vi "力特性判定.vi"(0 "曲线引用":refnum<vi>, 1 "力特性判定条件":T1, 3 "错误输入":errorcluster) -> (5 "曲线引用输出":refnum<vi>, 6 "OK？":bool, 8 "错误输出":errorcluster)   [LabVIEW 2019]
uses:
  Global_Variable/A131258.vi
  Global_Variable/Global.vi
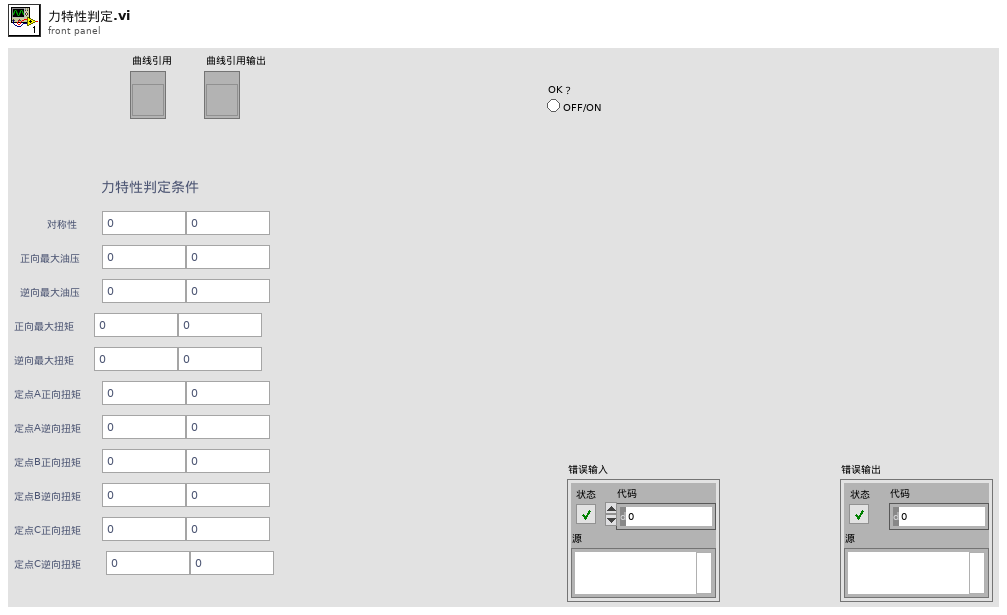
[diagram p1: front panel]
types:
  T1 = cluster{"           对称性":cluster{"下限":dbl, "上限":dbl}, "  正向最大油压":cluster{"下限":dbl, "上限":dbl}, "  逆向最大油压":cluster{"下限":dbl, "上限":dbl}, "正向最大扭矩":cluster{"下限":dbl, "上限":dbl}, "逆向最大扭矩":cluster{"下限":dbl, "上限":dbl}, "定点A正向扭矩":cluster{"下限":dbl, "上限":dbl}, "定点A逆向扭矩":cluster{"下限":dbl, "上限":dbl}, "定点B正向扭矩":cluster{"下限":dbl, "上限":dbl}, "定点B逆向扭矩":cluster{"下限":dbl, "上限":dbl}, "定点C正向扭矩":cluster{"下限":dbl, "上限":dbl}, "定点C逆向扭矩 ":cluster{"下限":dbl, "上限":dbl}}
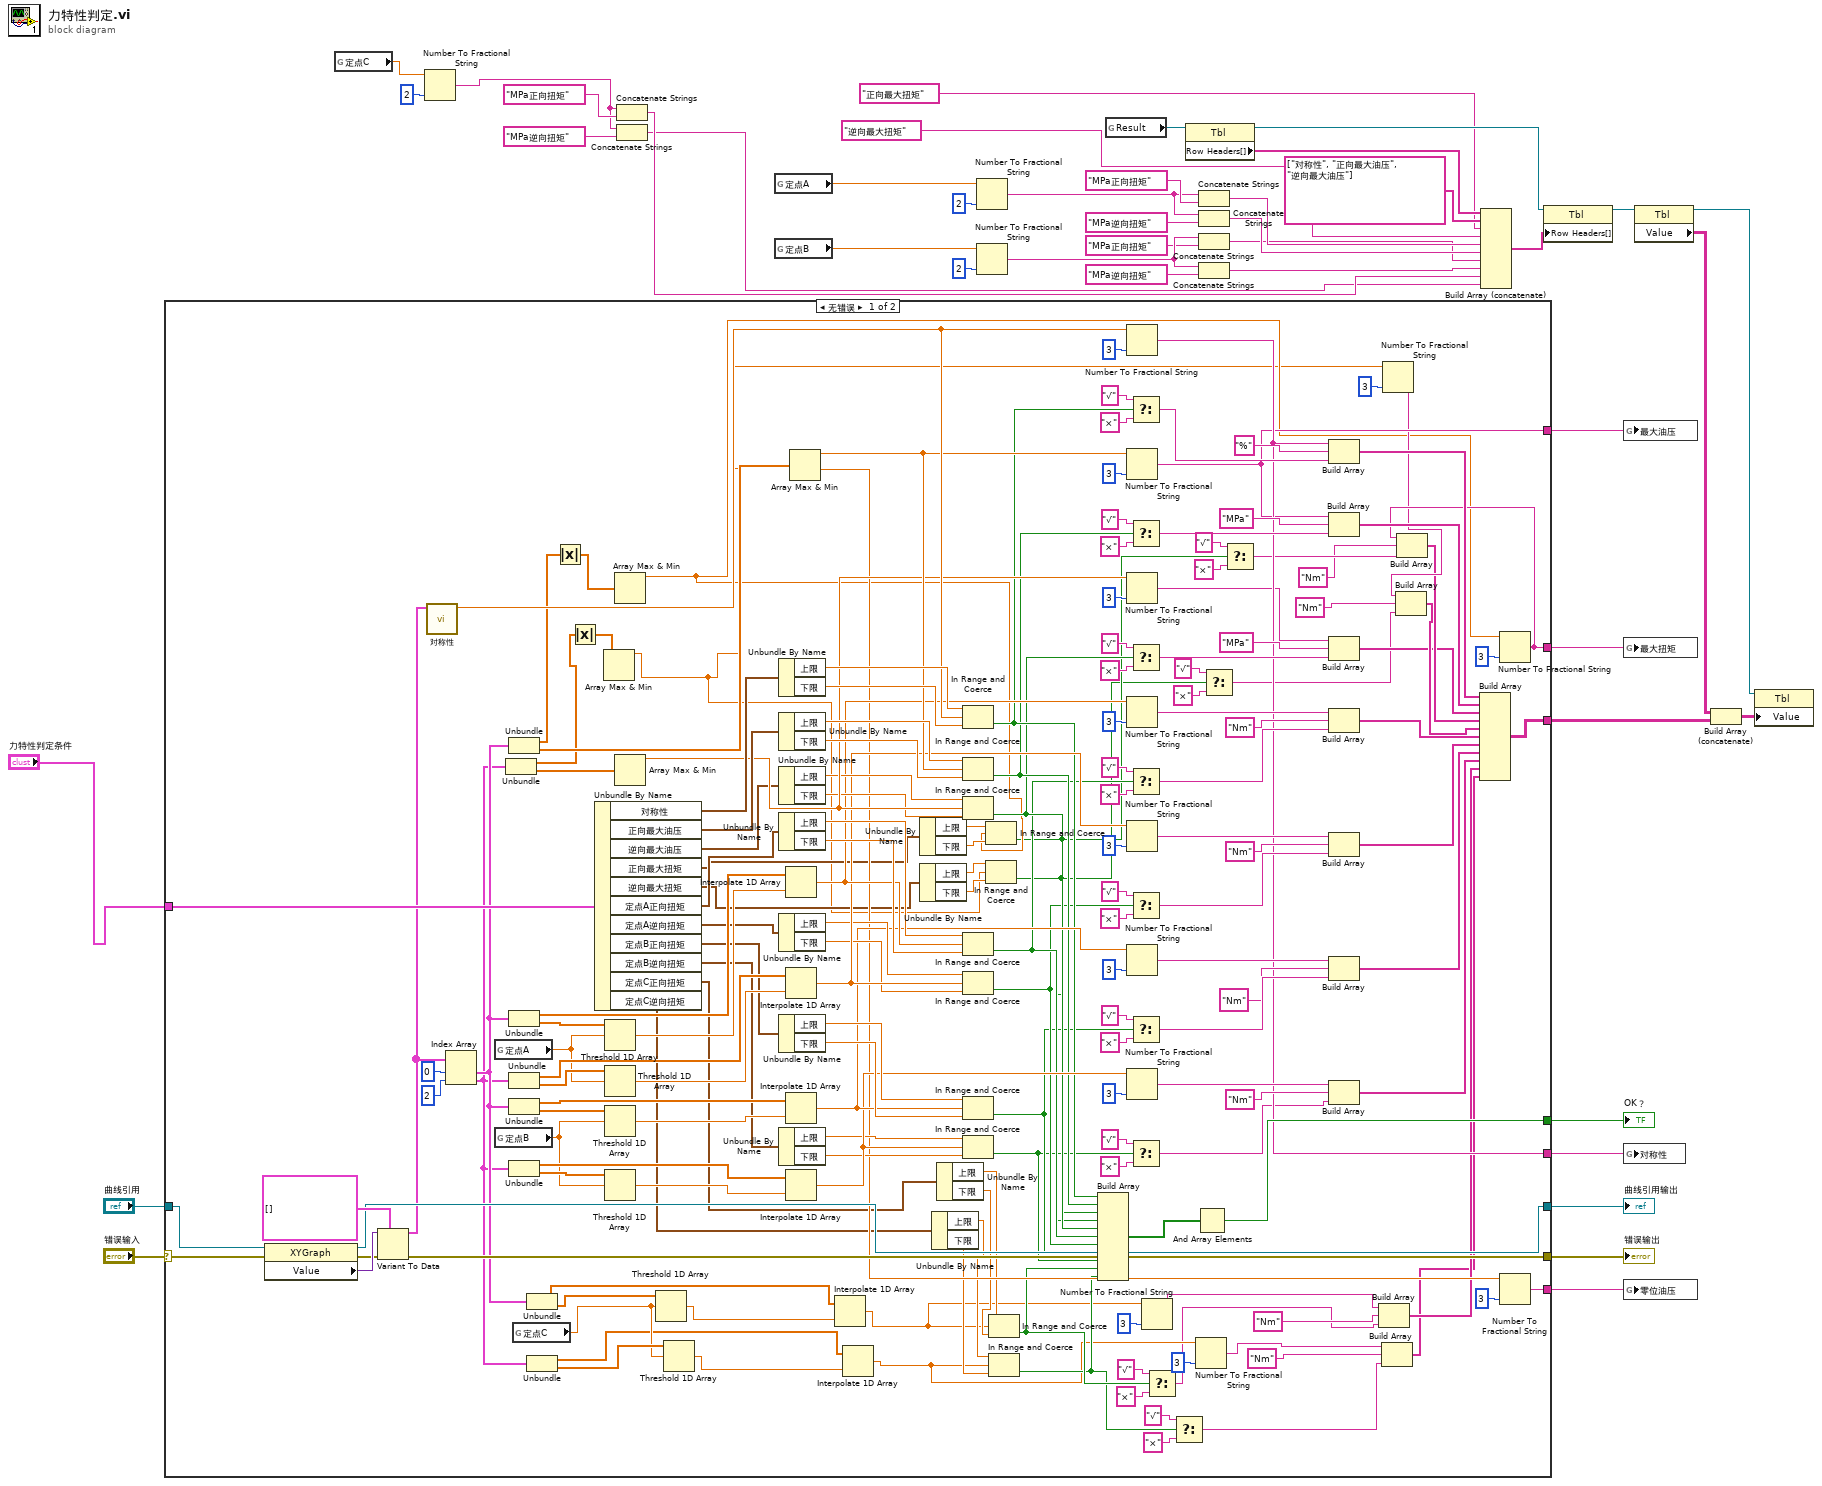
[diagram p0: block diagram]
diagram:
  n1 = case shown="无错误" "错误输入" {
    selector: "错误输入" -> [w219 w223]
    tunnel: [w216 w223] -> w42
    tunnel: "曲线引用" -> [w215 w222]
    tunnel: [w218 w222] -> w40
    tunnel: [w122 _] -> w39
    tunnel: "力特性判定条件" -> [w214 _]
    tunnel: [w121 _] -> w35
    tunnel: [w116 _] -> w14
    tunnel: [w115 _] -> w13
    tunnel: [w102 _] -> w12
    tunnel: [w111 _] -> w11
    frame No Error {
      n2 = property class="XYGraph"(reference=w215, error in=w219) -> (reference out=w218:refnum<vi>, error out=w217:errorcluster, "Value"=w221:variant)
      n3 = Variant To Data(error in=w217, type=cluster{dbl[], dbl[]}[] [], Variant=w221) -> (data=w204:cluster{dbl[], dbl[]}[], error out=w216:errorcluster)
      n4 = call "对称性.vi"("XY图"=w204) -> ("对称性"=w210:dbl)  [unwired: 8 in, 2 out]
      n5 = Index Array(array=w204, index #1=0 ("索引"), index #2=2 ("索引")) -> (element #1=w90:cluster{dbl[], dbl[]}, element #2=w89:cluster{dbl[], dbl[]})
      n6 = global read "A131258.vi" "定点A"() -> (w118:dbl)
      n7 = global read "A131258.vi" "定点B"() -> (w117:dbl)
      n8 = Unbundle(w89) -> (w47:dbl[], w119:dbl[])
      n9 = Unbundle(w90) -> (w45:dbl[], w120:dbl[])
      n10 = Unbundle(w90) -> (w176:dbl[], w177:dbl[])
      n11 = Unbundle(w89) -> (w171:dbl[], w170:dbl[])
      n12 = Unbundle(w90) -> (w152:dbl[], w153:dbl[])
      n13 = Unbundle(w89) -> (w145:dbl[], w144:dbl[])
      n14 = global read "A131258.vi" "定点C"() -> (w86:dbl)
      n15 = Unbundle(w90) -> (w83:dbl[], w88:dbl[])
      n16 = Unbundle(w89) -> (w82:dbl[], w87:dbl[])
      n17 = Absolute Value(x=w45) -> (abs(x)=w44:dbl[])
      n18 = Absolute Value(x=w47) -> (abs(x)=w48:dbl[])
      n19 = Unbundle By Name(w214) -> ("对称性"=w213:cluster{"下限":dbl, "上限":dbl}, "正向最大油压"=w196:cluster{"下限":dbl, "上限":dbl}, "逆向最大油压"=w186:cluster{"下限":dbl, "上限":dbl}, "正向最大扭矩"=w99:cluster{"下限":dbl, "上限":dbl}, "逆向最大扭矩"=w98:cluster{"下限":dbl, "上限":dbl}, "定点A正向扭矩"=w107:cluster{"下限":dbl, "上限":dbl}, "定点A逆向扭矩"=w108:cluster{"下限":dbl, "上限":dbl}, "定点B正向扭矩"=w109:cluster{"下限":dbl, "上限":dbl}, "定点B逆向扭矩"=w110:cluster{"下限":dbl, "上限":dbl}, "定点C正向扭矩"=w81:cluster{"下限":dbl, "上限":dbl}, "定点C逆向扭矩"=w80:cluster{"下限":dbl, "上限":dbl})
      n20 = Array Max & Min(array=w48) -> (max value=w46:dbl)  [unwired: 3 out]
      n21 = Threshold 1D Array(2:w118, 3:w177) -> (0:w175:dbl)  [unwired: 1 in]
      n22 = Threshold 1D Array(2:w118, 3:w170) -> (0:w172:dbl)  [unwired: 1 in]
      n23 = Threshold 1D Array(2:w117, 3:w153) -> (0:w151:dbl)  [unwired: 1 in]
      n24 = Threshold 1D Array(2:w117, 3:w144) -> (0:w146:dbl)  [unwired: 1 in]
      n25 = Array Max & Min(array=w44) -> (max value=w93:dbl)  [unwired: 3 out]
      n26 = Array Max & Min(array=w119) -> (max value=w194:dbl)  [unwired: 3 out]
      n27 = Threshold 1D Array(2:w86, 3:w88) -> (0:w85:dbl)  [unwired: 1 in]
      n28 = Threshold 1D Array(2:w86, 3:w87) -> (0:w84:dbl)  [unwired: 1 in]
      n29 = Unbundle By Name(w213) -> ("上限"=w212:dbl, "下限"=w211:dbl)
      n30 = Unbundle By Name(w196) -> ("上限"=w197:dbl, "下限"=w198:dbl)
      n31 = Unbundle By Name(w186) -> ("上限"=w193:dbl, "下限"=w192:dbl)
      n32 = Unbundle By Name(w107) -> ("上限"=w178:dbl, "下限"=w179:dbl)
      n33 = Unbundle By Name(w108) -> ("上限"=w169:dbl, "下限"=w168:dbl)
      n34 = Unbundle By Name(w109) -> ("上限"=w154:dbl, "下限"=w155:dbl)
      n35 = Unbundle By Name(w110) -> ("上限"=w143:dbl, "下限"=w142:dbl)
      n36 = Interpolate 1D Array(1:w175, 2:w176) -> (0:w174:dbl)
      n37 = Interpolate 1D Array(1:w172, 2:w171) -> (0:w173:dbl)
      n38 = Interpolate 1D Array(1:w151, 2:w152) -> (0:w150:dbl)
      n39 = Interpolate 1D Array(1:w146, 2:w145) -> (0:w147:dbl)
      n40 = Array Max & Min(array=w120) -> (max value=w195:dbl, min value=w112:dbl)  [unwired: 2 out]
      n41 = Interpolate 1D Array(1:w85, 2:w83) -> (0:w64:dbl)
      n42 = Interpolate 1D Array(1:w84, 2:w82) -> (0:w65:dbl)
      n43 = Unbundle By Name(w99) -> ("上限"=w97:dbl, "下限"=w96:dbl)
      n44 = Unbundle By Name(w98) -> ("上限"=w95:dbl, "下限"=w94:dbl)
      n45 = Unbundle By Name(w80) -> ("上限"=w77:dbl, "下限"=w76:dbl)
      n46 = Unbundle By Name(w81) -> ("上限"=w79:dbl, "下限"=w78:dbl)
      n47 = In Range and Coerce(upper limit=w212, x=w210, lower limit=w211) -> (In Range?=w135:bool)  [unwired: 1 out]
      n48 = In Range and Coerce(upper limit=w197, x=w195, lower limit=w198) -> (In Range?=w133:bool)  [unwired: 1 out]
      n49 = In Range and Coerce(upper limit=w193, x=w194, lower limit=w192) -> (In Range?=w132:bool)  [unwired: 1 out]
      n50 = In Range and Coerce(upper limit=w178, x=w174, lower limit=w179) -> (In Range?=w130:bool)  [unwired: 1 out]
      n51 = In Range and Coerce(upper limit=w169, x=w173, lower limit=w168) -> (In Range?=w128:bool)  [unwired: 1 out]
      n52 = In Range and Coerce(upper limit=w154, x=w150, lower limit=w155) -> (In Range?=w126:bool)  [unwired: 1 out]
      n53 = In Range and Coerce(upper limit=w143, x=w147, lower limit=w142) -> (In Range?=w124:bool)  [unwired: 1 out]
      n54 = In Range and Coerce(upper limit=w97, x=w93, lower limit=w96) -> (In Range?=w92:bool)  [unwired: 1 out]
      n55 = In Range and Coerce(upper limit=w95, x=w46, lower limit=w94) -> (In Range?=w91:bool)  [unwired: 1 out]
      n56 = In Range and Coerce(upper limit=w79, x=w64, lower limit=w78) -> (In Range?=w71:bool)  [unwired: 1 out]
      n57 = In Range and Coerce(upper limit=w77, x=w65, lower limit=w76) -> (In Range?=w70:bool)  [unwired: 1 out]
      n58 = Build Array(w135, w133, w92, w91, w132, w130, w128, w126, w124, w71, w70) -> (w123:bool[])
      n59 = Number To Fractional String(number=w210, precision (6)=i16 3 ("精度(6)")) -> (F-format string=w116:string)  [unwired: 2 in]
      n60 = Number To Fractional String(number=w195, precision (6)=i16 3 ("精度(6)")) -> (F-format string=w115:string)  [unwired: 2 in]
      n61 = Number To Fractional String(number=w194, precision (6)=i16 3 ("精度(6)")) -> (F-format string=w60:string)  [unwired: 2 in]
      n62 = Number To Fractional String(number=w174, precision (6)=i16 3 ("精度(6)")) -> (F-format string=w181:string)  [unwired: 2 in]
      n63 = Number To Fractional String(number=w173, precision (6)=i16 3 ("精度(6)")) -> (F-format string=w166:string)  [unwired: 2 in]
      n64 = Number To Fractional String(number=w150, precision (6)=i16 3 ("精度(6)")) -> (F-format string=w157:string)  [unwired: 2 in]
      n65 = Number To Fractional String(number=w147, precision (6)=i16 3 ("精度(6)")) -> (F-format string=w140:string)  [unwired: 2 in]
      n66 = Select(t="√" ("元素"), s=w135, f="×" ("元素")) -> (s? t:f=w205:string)
      n67 = Select(t="√" ("元素"), s=w133, f="×" ("元素")) -> (s? t:f=w203:string)
      n68 = Select(t="√" ("元素"), s=w132, f="×" ("元素")) -> (s? t:f=w187:string)
      n69 = Select(t="√" ("元素"), s=w130, f="×" ("元素")) -> (s? t:f=w185:string)
      n70 = Select(t="√" ("元素"), s=w128, f="×" ("元素")) -> (s? t:f=w162:string)
      n71 = Select(t="√" ("元素"), s=w126, f="×" ("元素")) -> (s? t:f=w161:string)
      n72 = Select(t="√" ("元素"), s=w124, f="×" ("元素")) -> (s? t:f=w49:string)
      n73 = Number To Fractional String(number=w64, precision (6)=i16 3 ("精度(6)")) -> (F-format string=w67:string)  [unwired: 2 in]
      n74 = Select(t="√" ("元素"), s=w71, f="×" ("元素")) -> (s? t:f=w50:string)
      n75 = Select(t="√" ("元素"), s=w70, f="×" ("元素")) -> (s? t:f=w52:string)
      n76 = Number To Fractional String(number=w65, precision (6)=i16 3 ("精度(6)")) -> (F-format string=w66:string)  [unwired: 2 in]
      n77 = And Array Elements(Boolean array=w123) -> (logical AND=w122:bool)
      n78 = Select(t="√" ("元素"), s=w91, f="×" ("元素")) -> (s? t:f=w54:string)
      n79 = Select(t="√" ("元素"), s=w92, f="×" ("元素")) -> (s? t:f=w57:string)
      n80 = Build Array(w116, "%" ("元素"), w205) -> (w136:string[])
      n81 = Build Array(w115, "MPa" ("元素"), w203) -> (w134:string[])
      n82 = Build Array(w60, "MPa" ("元素"), w187) -> (w61:string[])
      n83 = Build Array(w181, "Nm" ("元素"), w185) -> (w131:string[])
      n84 = Build Array(w166, "Nm" ("元素"), w162) -> (w129:string[])
      n85 = Build Array(w157, "Nm" ("元素"), w161) -> (w127:string[])
      n86 = Build Array(w140, "Nm" ("元素"), w49) -> (w125:string[])
      n87 = Build Array(w67, "Nm" ("元素"), w50) -> (w59:string[])
      n88 = Build Array(w66, "Nm" ("元素"), w52) -> (w58:string[])
      n89 = Number To Fractional String(number=w46, precision (6)=i16 3 ("精度(6)")) -> (F-format string=w100:string)  [unwired: 2 in]
      n90 = Build Array(w100, "Nm" ("元素"), w54) -> (w63:string[])
      n91 = Number To Fractional String(number=w93, precision (6)=i16 3 ("精度(6)")) -> (F-format string=w102:string)  [unwired: 2 in]
      n92 = Build Array(w102, "Nm" ("元素"), w57) -> (w62:string[])
      n93 = Build Array(w136, w134, w61, w62, w63, w131, w129, w127, w125, w59, w58) -> (w121:string[][])
      n94 = Number To Fractional String(number=w112, precision (6)=i16 3 ("精度(6)")) -> (F-format string=w111:string)  [unwired: 2 in]
    }
    frame Error {
    }
  }
  "错误输出" <- w42
  "曲线引用输出" <- w40
  "OK？" <- w39
  n95 = global read "A131258.vi" "定点C"() -> (w6:dbl)
  n96 = Number To Fractional String(number=w6, precision (6)=i16 2 ("精度(6)")) -> (F-format string=w3:string)  [unwired: 2 in]
  n97 = Concatenate Strings(w3, "MPa正向扭矩") -> (w2:string)
  n98 = Concatenate Strings(w3, "MPa逆向扭矩") -> (w1:string)
  n99 = global read "A131258.vi" "定点A"() -> (w28:dbl)
  n100 = global read "A131258.vi" "定点B"() -> (w27:dbl)
  n101 = Number To Fractional String(number=w28, precision (6)=i16 2 ("精度(6)")) -> (F-format string=w25:string)  [unwired: 2 in]
  n102 = Number To Fractional String(number=w27, precision (6)=i16 2 ("精度(6)")) -> (F-format string=w22:string)  [unwired: 2 in]
  n103 = global read "Global.vi" "Result"() -> (w34:refnum<vi>)
  n104 = property class="Tbl"(reference=w34) -> (reference out=w33:refnum<vi>, "Row Headers[]"=w31:string[])  [unwired: 1 in, 1 out]
  n105 = Concatenate Strings(w25, "MPa正向扭矩") -> (w20:string)
  n106 = Concatenate Strings(w25, "MPa逆向扭矩") -> (w19:string)
  n107 = Concatenate Strings(w22, "MPa正向扭矩") -> (w18:string)
  n108 = Concatenate Strings(w22, "MPa逆向扭矩") -> (w17:string)
  n109 = Build Array (concatenate)(w31, string[] ["对称性", "正向最大油压", "逆向最大油压"] ("列首字符串[]"), "正向最大扭矩", "逆向最大扭矩", w20, w19, w18, w17, w2, w1) -> (w29:string[])
  n110 = property class="Tbl"(reference=w33, "Row Headers[]"=w29) -> (reference out=w32:refnum<vi>)  [unwired: 1 in, 1 out]
  n111 = global write "检测结果.vi" "最大油压"(w13) -> ()
  n112 = global write "检测结果.vi" "最大扭矩"(w12) -> ()
  n113 = global write "检测结果.vi" "对称性"(w14) -> ()
  n114 = global write "检测结果.vi" "零位油压"(w11) -> ()
  n115 = property class="Tbl"(reference=w32) -> (reference out=w38:refnum<vi>, "Value"=w37:string[][])  [unwired: 1 in, 1 out]
  n116 = Build Array (concatenate)(w37, w35) -> (w36:string[][])
  n117 = property class="Tbl"(reference=w38, "Value"=w36) -> ()  [unwired: 1 in, 2 out]
